vi "init_exp_LF.vi"(0 "LightField Automation in":refnum<class "LightField Automation.lvclass">, 5 "Camera Choice":u16, 11 "error in (no error)":errorcluster) -> (2 "Array":cluster{"format string":string, string}[](array[cluster]), 3 "format string":string, 4 "LightField Automation out":refnum<class "LightField Automation.lvclass">, 6 "Visible":bool, 8 "Slit Width":dbl, 10 "Exposure Time (s)":dbl, 13 "Params CCD":string, 14 "ColumnCalibration":dbl[](array[numeric]), 15 "Center Wavelenght":dbl)   [LabVIEW 2019]
uses:
  lightfield-automation-labview/LightField Automation.lvclass
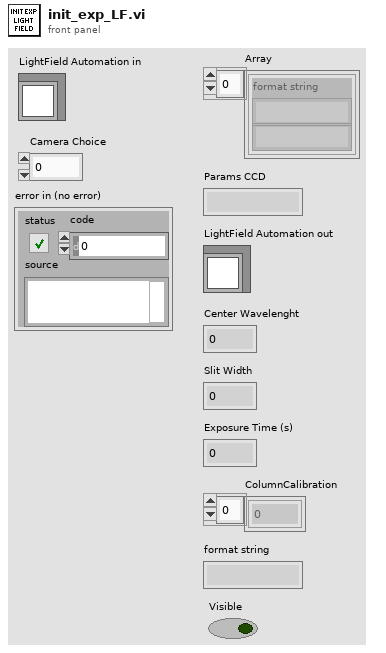
[diagram p1: front panel]
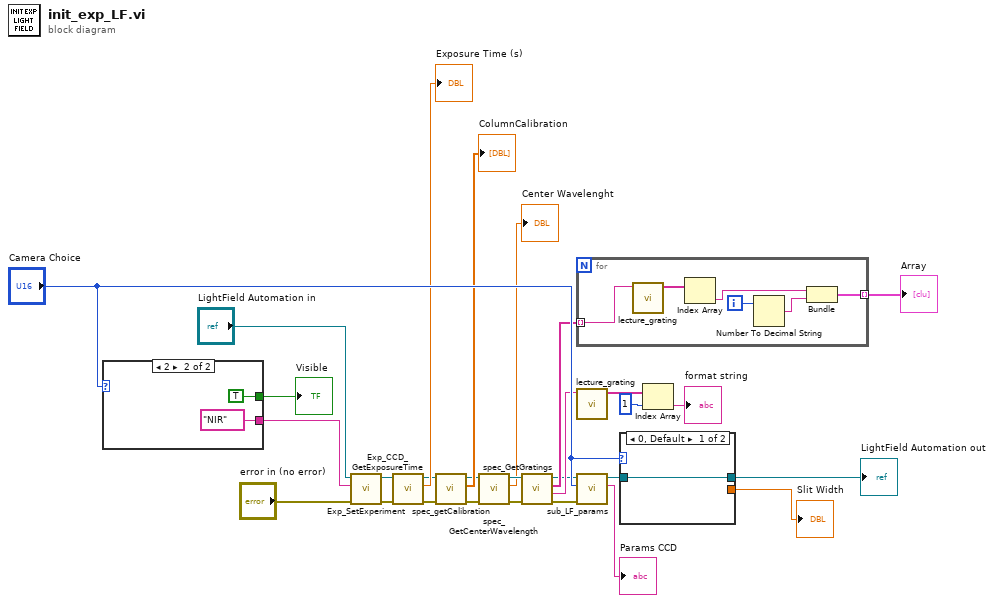
[diagram p0: block diagram]
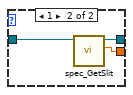
[diagram p2: hidden frame]
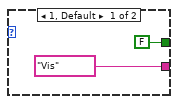
[diagram p3: hidden frame]
diagram:
  n1 = case shown="2" "Camera Choice" {
    tunnel: ["Vis" "NIR"] -> w3
    tunnel: [FALSE ("Visible") TRUE ("Visible")] -> w27
    frame 1, Default {
    }
    frame 2 {
    }
  }
  "Visible" <- w27
  n2 = call "Exp_SetExperiment.vi"("error in (no error)"="error in (no error)", "ExperimentName"=w3, "LightField Automation in"="LightField Automation in") -> ("error out"=w9:errorcluster, "LightField Automation out"=w6:refnum<class "LightField Automation.lvclass">)  [unwired: 7 in]
  n3 = call "Exp_CCD_GetExposureTime.vi"("error in (no error)"=w9, "LightField Automation in"=w6) -> ("error out"=w10:errorcluster, "Exposure Time (s)"=→"Exposure Time (s)":dbl, "LightField Automation out"=w7:refnum<class "LightField Automation.lvclass">)  [unwired: 7 in]
  n4 = call "spec_getCalibration.vi"("error in (no error)"=w10, "LightField Automation in"=w7) -> ("error out"=w11:errorcluster, "ColumnCalibration"=→"ColumnCalibration":dbl[], "LightField Automation out"=w8:refnum<class "LightField Automation.lvclass">)  [unwired: 7 in]
  n5 = call "spec_GetCenterWavelength.vi"("error in (no error)"=w11, "LightField Automation in"=w8) -> ("error out"=w5:errorcluster, "Center Wavelenght"=→"Center Wavelenght":dbl, "LightField Automation out"=w14:refnum<class "LightField Automation.lvclass">)  [unwired: 7 in]
  n6 = call "spec_GetGratings.vi"("error in (no error)"=w5, "LightField Automation in"=w14) -> ("error out"=w16:errorcluster, "Current Grating"=w20:string, "Gratings"=w18:string[], "LightField Automation out"=w15:refnum<class "LightField Automation.lvclass">)  [unwired: 6 in]
  n7 = for {
    tunnel: w18 -> [w38] mode=indexing
    tunnel: [w35] -> w19 mode=indexing
    i -> [w37]
    n8 = call "lecture_grating.vi"("GratingSelected"=w38) -> ("array"=w34:string[])  [unwired: 10 in]
    n9 = Index Array(array=w34) -> (element=w33:string)  [unwired: 1 in]
    n10 = Number To Decimal String(number=w37) -> (decimal integer string=w36:string)  [unwired: 1 in]
    n11 = Bundle("format string"=w33, w36) -> (w35:cluster{"format string":string, string})  [unwired: 1 in]
  }
  "Array" <- w19
  n12 = call "lecture_grating.vi"("GratingSelected"=w20) -> ("array"=w21:string[])  [unwired: 10 in]
  n13 = call "sub_LF_params.vi"("error in (no error)"=w16, "Numeric"="Camera Choice", "LightField Automation in"=w15) -> ("Params CCD"=→"Params CCD":string, "LightField Automation out"=w26:refnum<class "LightField Automation.lvclass">)  [unwired: 4 in, 1 out]
  n14 = case shown="0, Default" "Camera Choice" {
    tunnel: [w39 w41] -> w25
    tunnel: w26 -> [w39 w42]
    tunnel: [_ w40] -> w28
    frame 0, Default {
    }
    frame 1 {
      n15 = call "spec_GetSlit.vi"("LightField Automation in"=w42) -> ("Slit Width"=w40:dbl, "LightField Automation out"=w41:refnum<class "LightField Automation.lvclass">)  [unwired: 8 in, 1 out]
    }
  }
  "Slit Width" <- w28
  "LightField Automation out" <- w25
  n16 = Index Array(array=w21, index=1) -> (element=→"format string":string)
